vi "dfd_Extract Header to Get Filter String.vi"(11 "string in":string) -> (3 "string out":string)   [LabVIEW 2017, in "NI_DigFilter_Process.lvlib"]
uses:
  <vilib>/addons/Digital Filter Design/NI_DigFilter_Process.lvlib
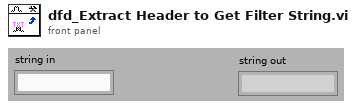
[diagram p1: front panel]
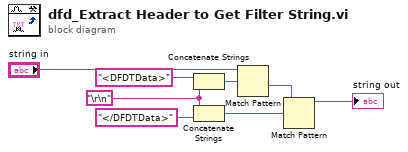
[diagram p0: block diagram]
diagram:
  w3 = "\r\n"
  n1 = Concatenate Strings("<DFDTData>", w3) -> (w4:string)
  n2 = Concatenate Strings(w3, "</DFDTData>" ("Substring")) -> (w5:string)
  n3 = Match Pattern(string="string in", regular expression=w4) -> (after substring=w6:string)  [unwired: 4 out]
  n4 = Match Pattern(string=w6, regular expression=w5) -> (before substring=→"string out":string)  [unwired: 4 out]
